vi "GetAllPendingData.vi"(8 "error in (no error)":errorcluster, 11 "config":T1) -> (0 "error out":errorcluster, 3 "all pending data":variant[](array[variant]))   [LabVIEW 2017, in "FileManager.lvlib"]
uses:
  <vilib>/addons/InsightCM/Devices/Shared/Common/FileManager/FileManager.lvlib
  <vilib>/addons/InsightCM/Devices/Shared/Common/FileManager/controls/config.ctl
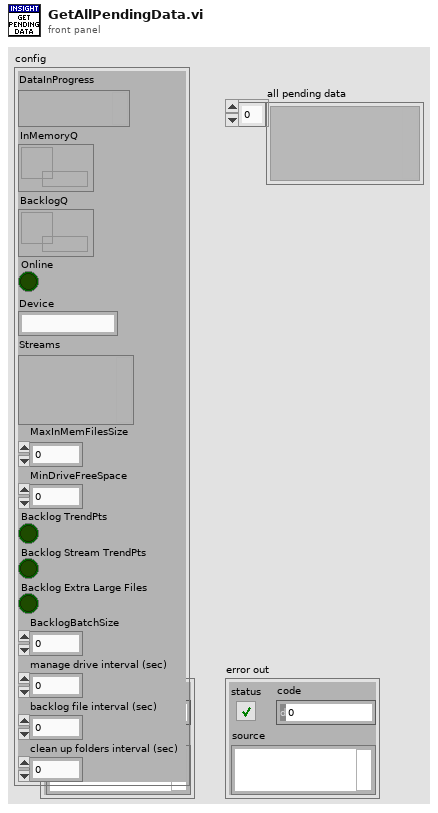
[diagram p1: front panel]
types:
  T1 = typedef "FileManager.lvlib/config.ctl" = cluster{"DataInProgress":variant, "InMemoryQ":refnum<queue>, "BacklogQ":refnum<queue>, "Online":bool, "Device":string, "Streams":variant, "MaxInMemFilesSize":i32, "MinDriveFreeSpace":i32, "Backlog TrendPts":bool, "Backlog Stream TrendPts":bool, "Backlog Extra Large Files":bool, "BacklogBatchSize":i32, "manage drive interval (sec)":dbl, "backlog file interval (sec)":dbl, "clean up folders interval (sec)":dbl}
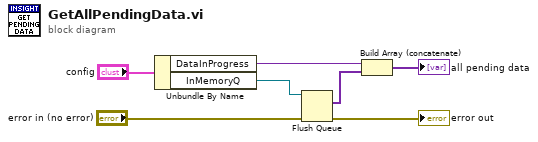
[diagram p0: block diagram]
diagram:
  n1 = Unbundle By Name("config") -> ("DataInProgress"=w4:variant, "InMemoryQ"=w5:refnum<queue>)
  n2 = Flush Queue(queue=w5, error in (no error)="error in (no error)") -> (remaining elements=w3:variant[], error out=→"error out":errorcluster)  [unwired: 1 out]
  n3 = Build Array (concatenate)(w4, w3) -> (→"all pending data":variant[])
